vi "FlexDDS-NG_DCP_WriteDRR.vi"(8 "digital ramp positive slope rate":u16=100, 9 "digital ramp negative slope rate":u16=100, 10 "Channels":T1(ring)=enum."Both channels", 11 "initial instruction string":string) -> (3 "appended instruction string":string="dcp spi:DRR=0x640064\r")   [LabVIEW 2016]
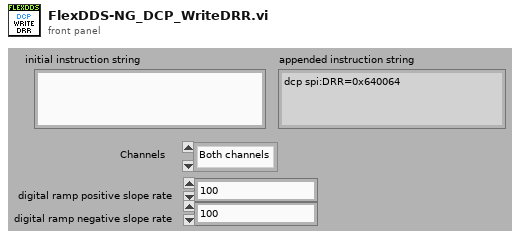
[diagram p1: front panel]
types:
  T1 = enum32{"Channel 0", "Channel 1", "Both channels"}
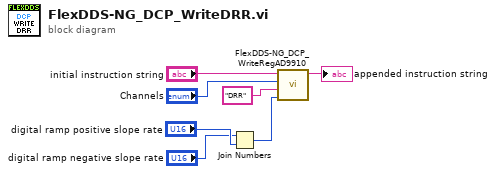
[diagram p0: block diagram]
diagram:
  n1 = Join Numbers(hi="digital ramp negative slope rate", lo="digital ramp positive slope rate") -> ((hi.lo)=w3:u32)
  n2 = call "FlexDDS-NG_DCP_WriteRegAD9910.vi"("register content"=w3, "AD9910 register name"="DRR" ("format string"), "Channels"="Channels", "initial instruction string"="initial instruction string") -> ("appended instruction string"=→"appended instruction string":string)  [unwired: 7 in]
